vi "Programmer.vi"(0 "Number of Repetitions":i32, 1 "Action":T7=enum."Execute Programmer", 5 "Step Array":T5[](array[typedef])=[{"Airflow (CFM)"={"Setpoint"=0.0, "Stability Range (±)"=0.0}, "Air Temp (°F)"={"Setpoint"=0.0, "Stability Range (±)"=0.0}, "Glycol Flow (lbm/hr)"={"Setpoint"=0.0, "Stability Range (±)"=0.0}, "Glycol Temp (°F)"={"Setpoint"=0.0, "Stability Range (±)"=0.0}, "Hold Time (min)"=0.0, "Stability Test Time (min)"=0.0, "Stability Timeout (min)"=0.0, "Defrost?"=FALSE}], 9 "ANALOG In":T2, 11 "error in (no error)":errorcluster, 12 "Calc Values In":T3) -> (2 "Defrost?":bool, 3 "Setpoints":T4, 4 "Testing is Active?":bool=TRUE, 6 "Current Step":i32, 8 "Time til Step End":dbl format="%<%H:%M:%S>t", 10 "Programmer State":T1, 14 "Components Stable?":bool[](array[boolean]), 15 "error out":errorcluster)   [LabVIEW 2012]
uses:
  Data Types/Programmer Execution States.ctl
  Data Types/Programmer Step.ctl
  Data Types/Programmer Step References.ctl
  Controls/HXG2_Calculated.ctl
  Controls/HXG2_AnalogIn.ctl
  Data Types/Programmer State.ctl
  Support/Time Based Queue/TimeBasedQueue.lvclass
  HXG2programmer.ctl
panel:
  in  "User Input Cluster":T4
  # "Stability (min)"
  # "Running (min)"
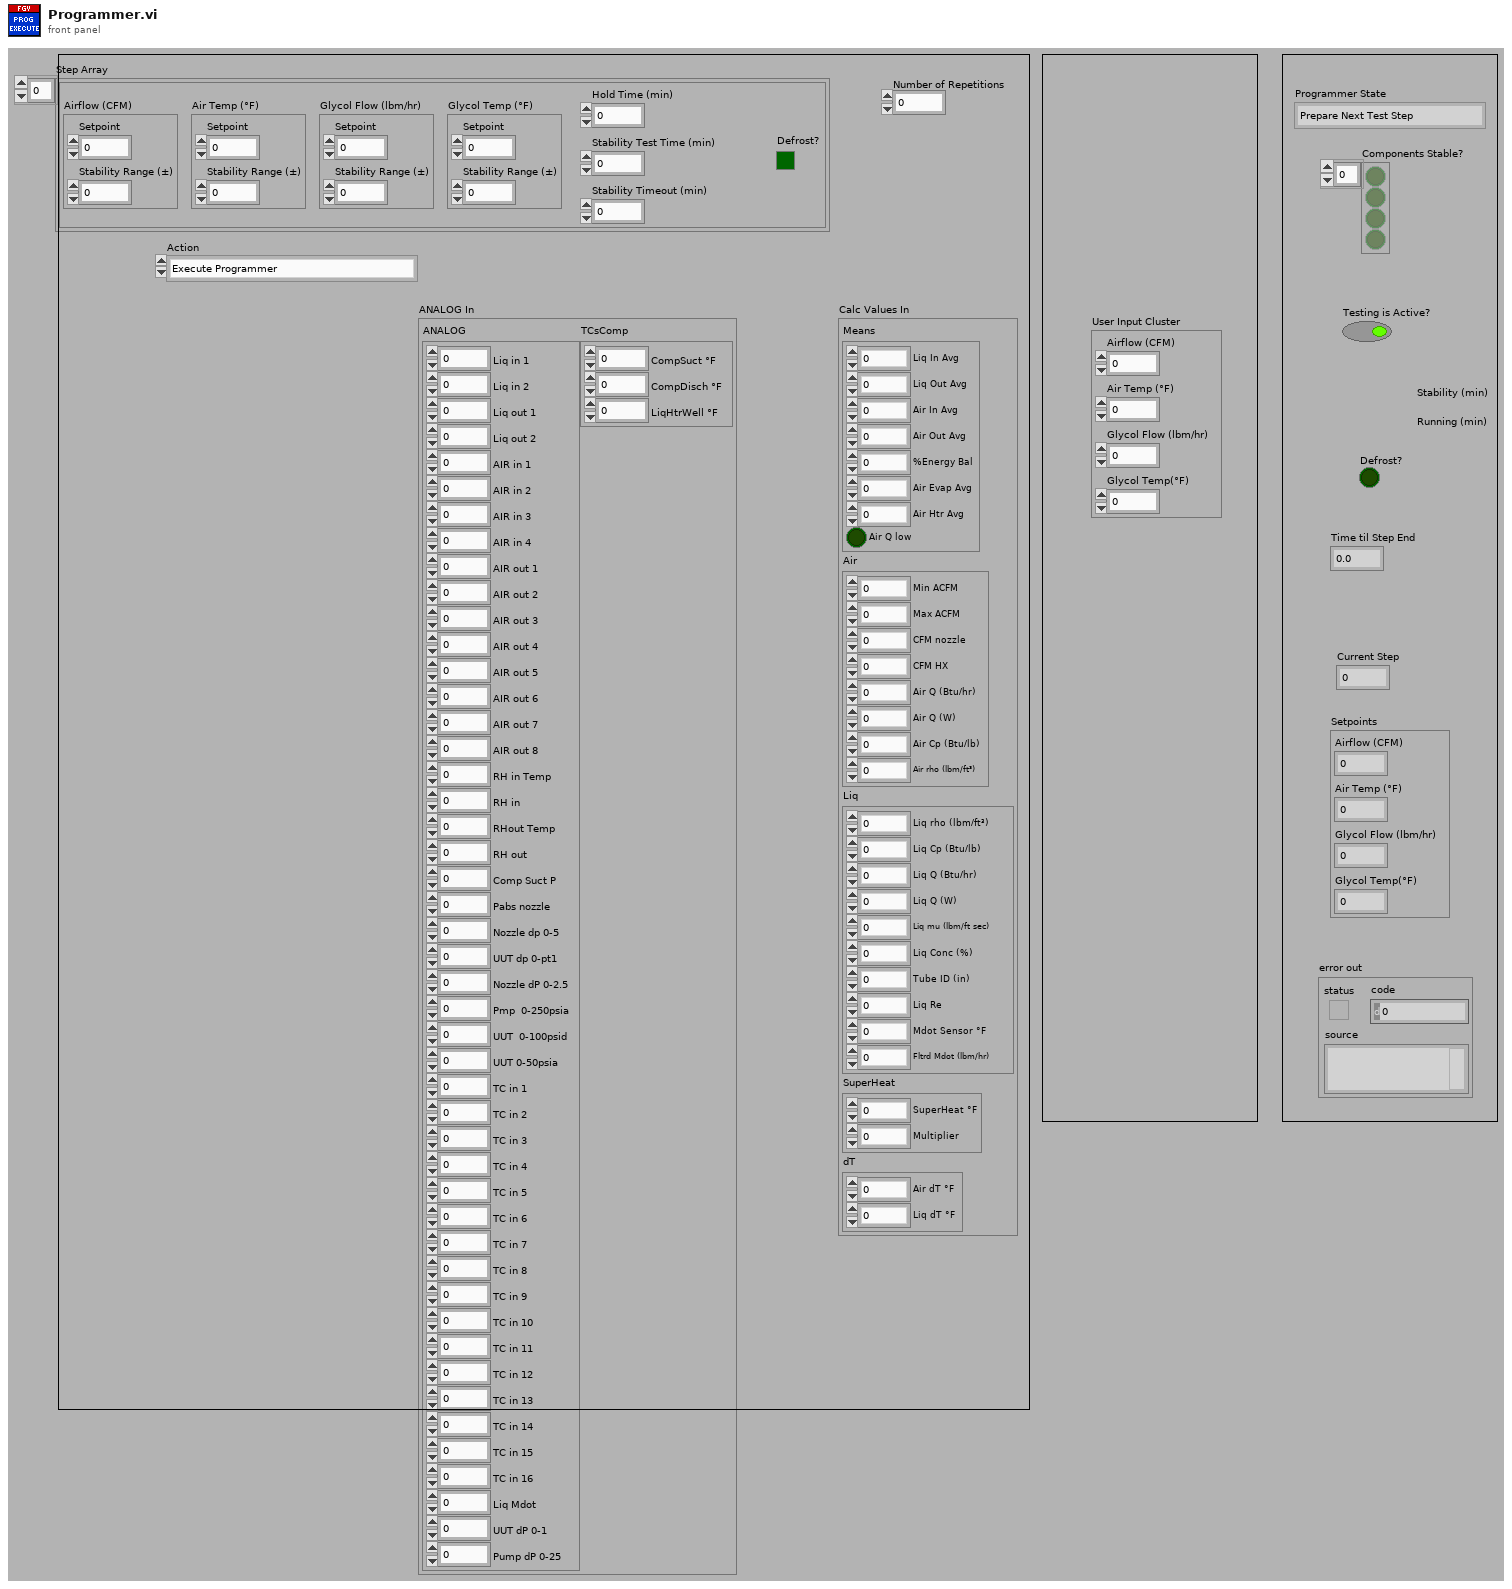
[diagram p1: front panel]
types:
  T1 = typedef "Programmer State.ctl" = enum16{"Prepare Next Test Step", "Stopped", "Running", "Stabilizing"}
  T2 = typedef "HXG2_AnalogIn.ctl" = cluster{"ANALOG":cluster{"Liq in 1":dbl, "Liq in 2":dbl, "Liq out 1":dbl, "Liq out 2":dbl, "AIR in 1":dbl, "AIR in 2":dbl, "AIR in 3":dbl, "AIR in 4":dbl, "AIR out 1":dbl, "AIR out 2":dbl, "AIR out 3":dbl, "AIR out 4":dbl, "AIR out 5":dbl, "AIR out 6":dbl, "AIR out 7":dbl, "AIR out 8":dbl, "RH in Temp":dbl, "RH in":dbl, "RHout Temp":dbl, "RH out":dbl, "Comp Suct P":dbl, "Pabs nozzle":dbl, "Nozzle dp 0-5":dbl, "UUT dp 0-pt1":dbl, "Nozzle dP 0-2.5":dbl, "Pmp  0-250psia":dbl, "UUT  0-100psid":dbl, "UUT 0-50psia":dbl, "TC in 1":dbl, "TC in 2":dbl, "TC in 3":dbl, "TC in 4":dbl, "TC in 5":dbl, "TC in 6":dbl, "TC in 7":dbl, "TC in 8":dbl, "TC in 9":dbl, "TC in 10":dbl, "TC in 11":dbl, "TC in 12":dbl, "TC in 13":dbl, "TC in 14":dbl, "TC in 15":dbl, "TC in 16":dbl, "Liq Mdot":dbl, "UUT dP 0-1":dbl, "Pump dP 0-25":dbl}, "TCsComp":cluster{"CompSuct °F  ":dbl, "CompDisch °F":dbl, "LiqHtrWell °F":dbl}}
  T3 = typedef "HXG2_Calculated.ctl" = cluster{"Means":cluster{"Liq In Avg":dbl, "Liq Out Avg":dbl, "Air In Avg":dbl, "Air Out Avg":dbl, "%Energy Bal":dbl, "Air Evap Avg":dbl, "Air Htr Avg":dbl, "Air Q low":bool}, "Air":cluster{"Min ACFM":dbl, "Max ACFM":dbl, "CFM nozzle":dbl, "CFM HX":dbl, "Air Q (Btu/hr)":dbl, "Air Q (W)":dbl, "Air Cp (Btu/lb)":dbl, "Air rho (lbm/ft³)":dbl}, "Liq":cluster{"Liq rho (lbm/ft³)":dbl, "Liq Cp (Btu/lb)":dbl, "Liq Q (Btu/hr)":dbl, "Liq Q (W)":dbl, "Liq mu (lbm/ft sec)":dbl, "Liq Conc (%)":dbl, "Tube ID (in)":dbl, "Liq Re":dbl, "Mdot Sensor °F":dbl, "Fltrd Mdot (lbm/hr)":dbl}, "SuperHeat":cluster{"SuperHeat °F":dbl, "Multiplier":dbl}, "dT":cluster{"Air dT °F":dbl, "Liq dT °F":dbl}}
  T4 = cluster{"Airflow (CFM)":dbl, "Air Temp (°F)":dbl, "Glycol Flow (lbm/hr)":dbl, "Glycol Temp(°F)":dbl}
  T5 = typedef "Programmer Step.ctl" = cluster{"Airflow (CFM)":T6, "Air Temp (°F)":T6, "Glycol Flow (lbm/hr)":T6, "Glycol Temp (°F)":T6, "Hold Time (min)":dbl, "Stability Test Time (min)":dbl, "Stability Timeout (min)":dbl, "Defrost?":bool}
  T6 = typedef "Programmer Step References.ctl" = cluster{"Setpoint":dbl, "Stability Range (±)":dbl}
  T7 = typedef "Programmer Execution States.ctl" = enum16{"Register Steps", "Initialize", "Start Test Sequence", "Register Data", "Execute Programmer", "Set Number of Repetitions", "Get Current Step Index", "Get Time Until Step Ends"}
  T8 = typedef "HXG2programmer.ctl" = enum16{"Write Refs", "Write Selec", "Write All", "Pass All", "React", "Write Path"}
  T9 = typedef "HXG2_ProgRefs.ctl" = cluster{"Prog. Indicator":refnum<vi>, "Table":refnum<vi>, "Save Button":refnum<vi>, "Duration Ctrl":refnum<vi>, "Run Prog":refnum<vi>}
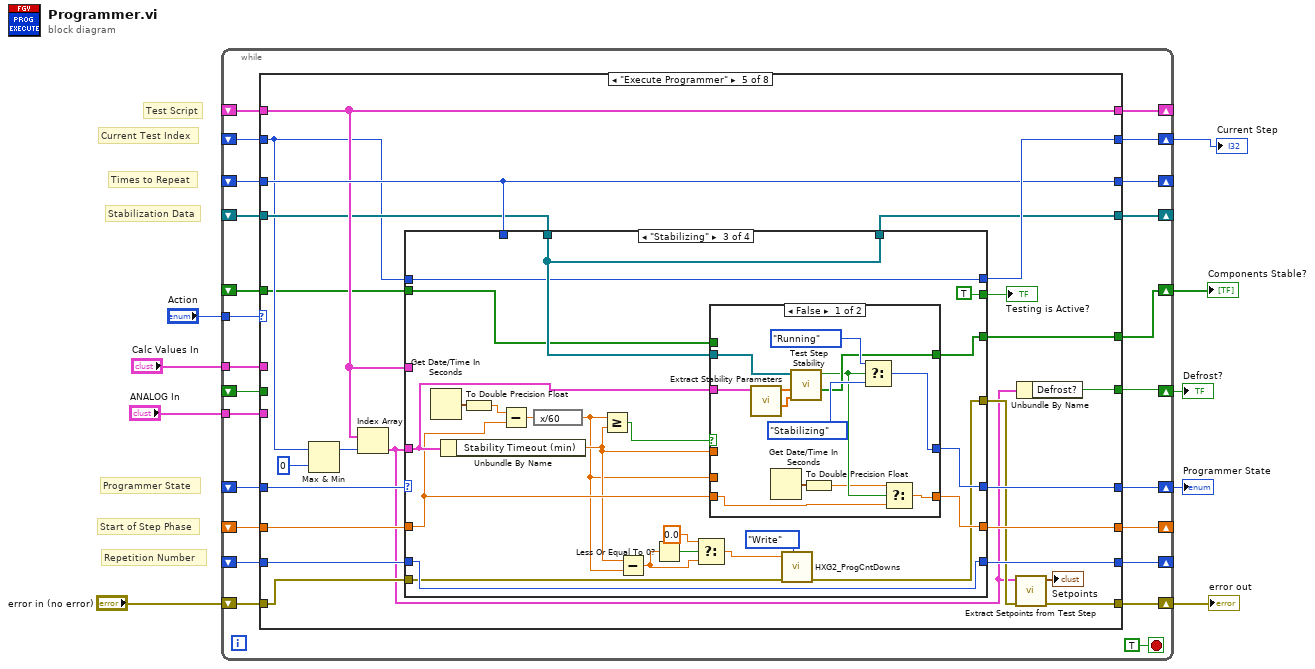
[diagram p0: block diagram]
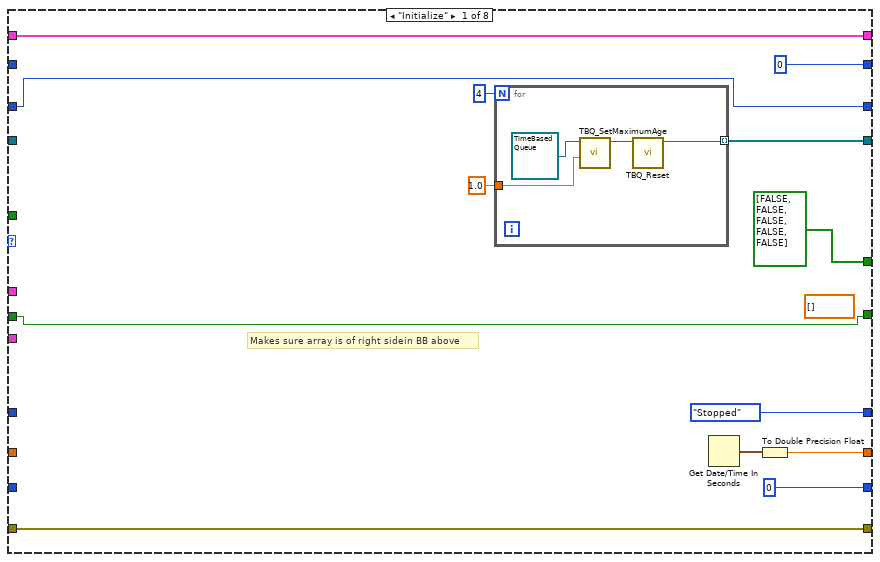
[diagram p2: hidden frame]
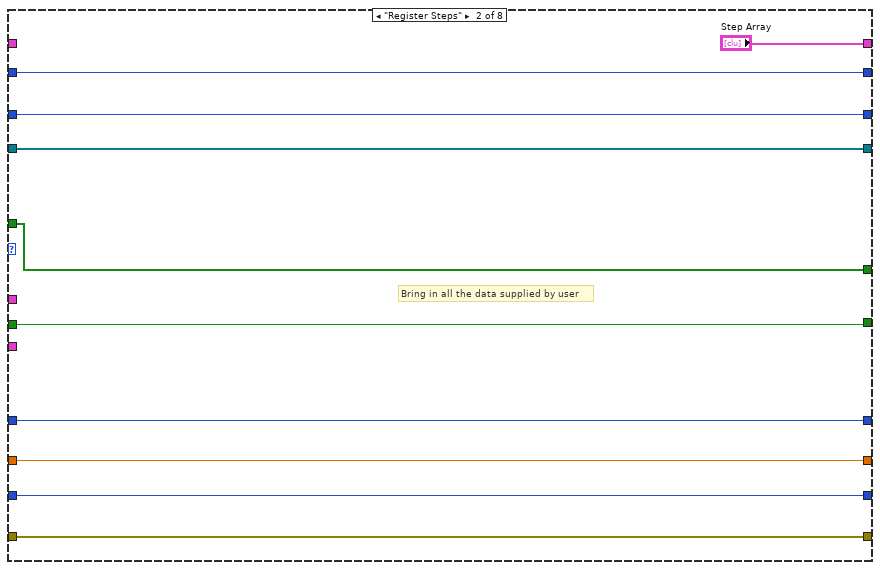
[diagram p3: hidden frame]
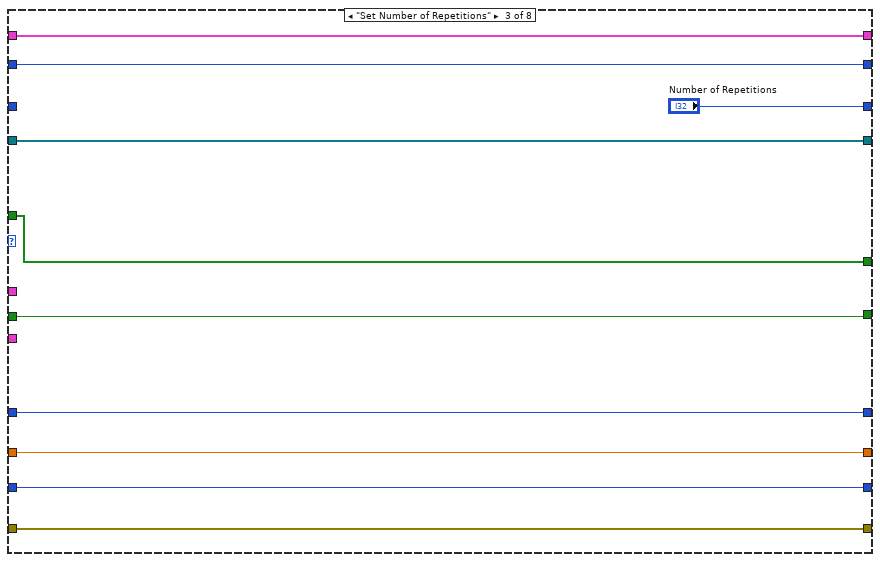
[diagram p4: hidden frame]
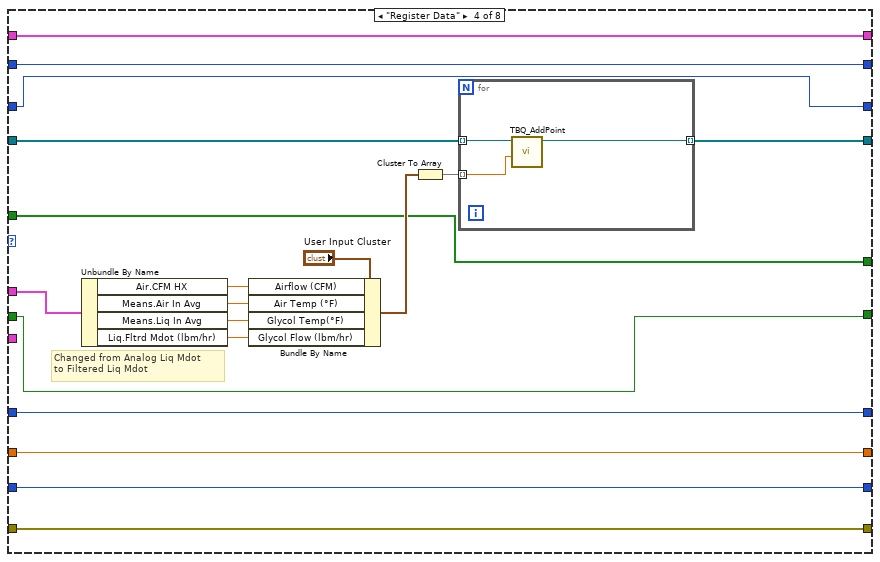
[diagram p5: hidden frame]
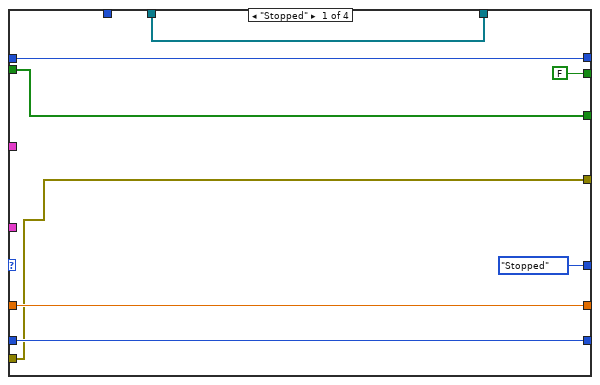
[diagram p6: hidden frame]
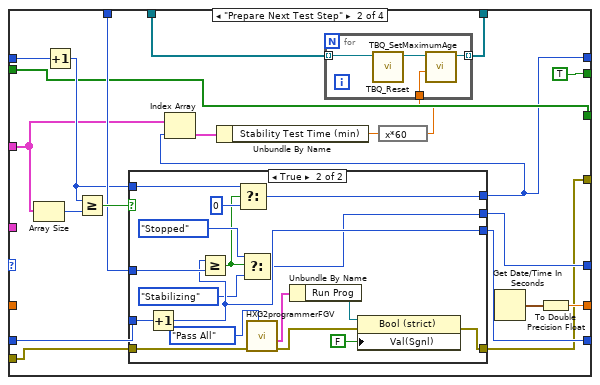
[diagram p7: hidden frame]
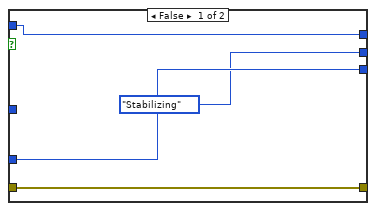
[diagram p8: hidden frame]
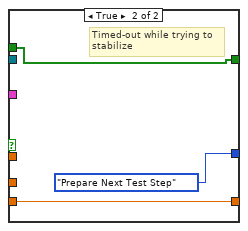
[diagram p9: hidden frame]
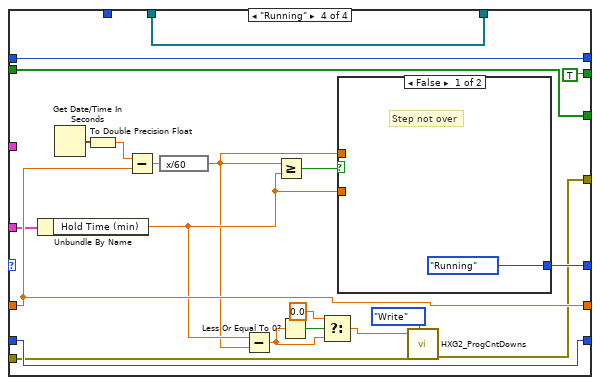
[diagram p10: hidden frame]
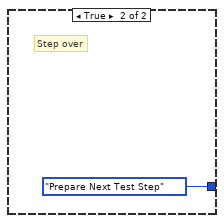
[diagram p11: hidden frame]
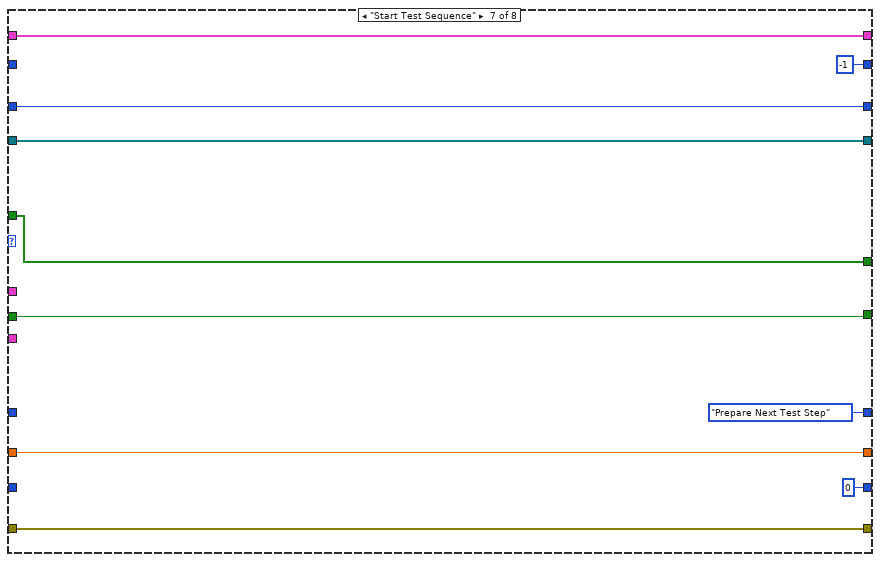
[diagram p13: hidden frame]
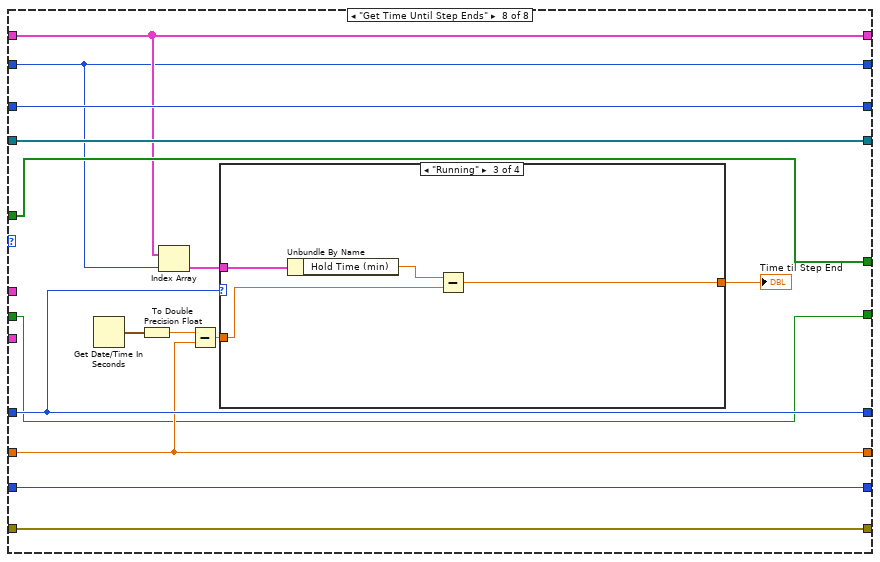
[diagram p14: hidden frame]
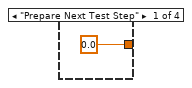
[diagram p15: hidden frame]
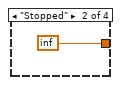
[diagram p16: hidden frame]
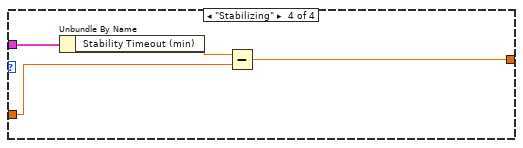
[diagram p17: hidden frame]
diagram:
  # "Repetition Number"
  # "Times to Repeat"
  # "Start of Step Phase"
  # "Programmer State"
  # "Stabilization Data"
  # "Current Test Index"
  # "Test Script"
  n1 = while {
    tunnel: "Action" -> [w33]
    shift-right: [w32] -> _
    shift-left: _ -> [w31]
    shift-right: [w29] -> w2
    shift-left: _ -> [w28]
    shift-right: [w27] -> w8
    shift-left: "error in (no error)" -> [w26]
    shift-right: [w25] -> _
    shift-left: _ -> [w24]
    shift-right: [w23] -> w4
    shift-left: _ -> [w22]
    shift-right: [w21] -> _
    shift-left: _ -> [w20]
    shift-right: [w19] -> _
    shift-left: _ -> [w18]
    shift-right: [w17] -> _
    shift-left: _ -> [w16]
    tunnel: "ANALOG In" -> [w15]
    tunnel: "Calc Values In" -> [w14]
    shift-right: [w13] -> w3
    shift-left: _ -> [w12]
    shift-right: [w11] -> w1
    shift-left: _ -> [w10]
    stop <- TRUE stop-if-true
    n2 = case shown="\"Execute Programmer\"" w33 {
      tunnel: [w42 "Step Array" w70 w89 w106 w241 w251 w256] -> w32
      tunnel: w31 -> [w42 _ w70 w89 w106 w241 w251 w256]
      tunnel: [0 w59 w69 w88 w113 w233 -1 ("f") w255] -> w29
      tunnel: w28 -> [_ w59 w69 w88 w100 w233 _ w255]
      tunnel: [w45 w58 w68 w87 w104 w240 w250 w266] -> w27
      tunnel: w26 -> [w45 w58 w68 w87 w96 w240 w250 w266]
      tunnel: [w44 w57 w67 w84 w102 w239 w249 w265] -> w25
      tunnel: w24 -> [_ w57 w67 w85 w103 w239 w249 w265]
      tunnel: [Programmer_State."Stopped" ("Programmer State") w55 w66 w82 w112 w237 Programmer_State."Prepare Next Test Step" ("Programmer State") w254] -> w23
      tunnel: w22 -> [_ w55 w66 w82 w115 w237 _ w254]
      tunnel: [w40 w56 w65 w83 w111 w238 w248 w253] -> w21
      tunnel: w20 -> [_ w56 w65 w83 w114 w238 w248 w253]
      tunnel: [w38 w54 "Number of Repetitions" w81 w109 w236 w247 w264] -> w19
      tunnel: w18 -> [w38 w54 _ w81 w109 w236 w247 w264]
      tunnel: [0 w53 w63 w80 w108 w235 0 w263] -> w17
      tunnel: w16 -> [_ w53 w63 w80 w110 w235 _ w263]
      tunnel: w15 -> [_ _ _ _ _ _ _ _]
      tunnel: w14 -> [_ _ _ w77 _ _ _ _]
      tunnel: [bool[] [FALSE, FALSE, FALSE, FALSE, FALSE] ("Components Stable?") w52 w62 w73 w98 w234 w243 w262] -> w13
      tunnel: w12 -> [_ w52 w62 w73 w97 w234 w243 w262]
      tunnel: [w34 w51 w61 w71 w93 w232 w242 w252] -> w11
      tunnel: w10 -> [w34 w51 w61 w71 _ w232 w242 w252]
      frame "Initialize" {
        (unwired) dbl[] []
        # "Makes sure array is of right sidein BB above"
        n3 = for {
          N: 4 -> [_]
          tunnel: [w48] -> w44 mode=indexing
          tunnel: 1.0 ("Stability Test Time (min)") -> [w47]
          n4 = call "TBQ_SetMaximumAge.vi"("Maximum Age (s)"=w47, "TimeBasedQueue In"=refnum<class "TimeBasedQueue.lvclass"> refnum ("TimeBasedQueue.lvclass")) -> ("TimeBasedQueue Out"=w49:refnum<class "TimeBasedQueue.lvclass">)  [unwired: 9 in]
          n5 = call "TBQ_Reset.vi"("TimeBasedQueue In"=w49) -> ("TimeBasedQueue Out"=w48:refnum<class "TimeBasedQueue.lvclass">)  [unwired: 10 in]
        }
        n6 = Get Date/Time In Seconds() -> (seconds since 1Jan1904=w41:timestamp)
        n7 = To Double Precision Float(number=w41) -> (double precision float=w40:dbl)
      }
      frame "Register Steps" {
        # "Bring in all the data supplied by user"
      }
      frame "Set Number of Repetitions" {
      }
      frame "Register Data" {
        # "Changed from Analog Liq Mdot\nto Filtered Liq Mdot"
        n8 = Unbundle By Name(w77) -> ("Air.CFM HX"=w76:dbl, "Means.Air In Avg"=w75:dbl, "Means.Liq In Avg"=w74:dbl, "Liq.Fltrd Mdot (lbm/hr)"=w72:dbl)
        n9 = Bundle By Name(cluster="User Input Cluster", "Airflow (CFM)"=w76, "Air Temp (°F)"=w75, "Glycol Temp(°F)"=w74, "Glycol Flow (lbm/hr)"=w72) -> (w79:T4)
        n10 = Cluster To Array(cluster=w79) -> (array=w86:dbl[])
        n11 = for {
          tunnel: w86 -> [w91] mode=indexing
          tunnel: w85 -> [w92] mode=indexing
          tunnel: [w90] -> w84 mode=indexing
          n12 = call "TBQ_AddPoint.vi"("New Data Point"=w91, "TimeBasedQueue In"=w92) -> ("TimeBasedQueue Out"=w90:refnum<class "TimeBasedQueue.lvclass">)  [unwired: 9 in]
        }
      }
      frame "Execute Programmer" {
        n13 = Max & Min(x=w100, y=0) -> (max(x,y)=w99:i32)  [unwired: 1 out]
        n14 = Index Array(array=w106, index=w99) -> (element=w94:T5)
        n15 = case shown="\"Stabilizing\"" w115 {
          tunnel: w103 -> [w118 w130 w192 w219]
          tunnel: [Programmer_State."Stopped" ("Programmer State") w136 w191 w225] -> w112
          tunnel: w114 -> [w120 _ w179 w223]
          tunnel: w94 -> [_ _ w186 w220]
          tunnel: w100 -> [w122 w142 w185 w224]
          tunnel: [w122 w126 w185 w224] -> w113
          tunnel: [w120 w143 w180 w223] -> w111
          tunnel: w110 -> [w123 w139 w184 w222]
          tunnel: w106 -> [_ w133 _ _]
          tunnel: w109 -> [_ w138 _ _]
          tunnel: [w123 w137 w184 w222] -> w108
          tunnel: [FALSE TRUE TRUE TRUE] -> w107
          tunnel: [w118 w129 w192 w219] -> w102
          tunnel: [w117 w128 w182 w218] -> w98
          tunnel: w97 -> [w117 w128 w181 w218]
          tunnel: w96 -> [w116 w125 w175 w212]
          tunnel: [w116 w124 w174 w211] -> w95
          frame "Stopped" {
          }
          frame "Prepare Next Test Step" {
            n16 = Array Size(array=w133) -> (size(s)=w140:i32)
            n17 = Increment(x=w142) -> (x+1=w135:i32)
            n18 = Greater Or Equal?(x=w135, y=w140) -> (x >= y?=w141:bool)
            n19 = case shown="True" w141 {
              tunnel: w139 -> [w152 w169]
              tunnel: w138 -> [_ w168]
              tunnel: [w152 w167] -> w137
              tunnel: [Programmer_State."Stabilizing" ("Programmer State") w166] -> w136
              tunnel: w135 -> [w150 w163]
              tunnel: [w150 w162] -> w126
              tunnel: w125 -> [w149 w154]
              tunnel: [w149 w153] -> w124
              frame False {
              }
              frame True {
                n20 = Increment(x=w169) -> (x+1=w167:i32)
                n21 = Greater Or Equal?(x=w167, y=w168) -> (x >= y?=w160:bool)
                n22 = Select(t=w163, s=w160, f=0) -> (s? t:f=w162:i32)
                n23 = Select(t=Programmer_State."Stopped" ("Programmer State"), s=w160, f=Programmer_State."Stabilizing" ("Programmer State")) -> (s? t:f=w166:T1)
                n24 = call "HXG2programmerFGV.vi"("Programmer Ctrl"=HXG2programmer."Pass All", "error in (no error)"=w154) -> ("error out"=w158:errorcluster, "References Out"=w156:T9)  [unwired: 5 in, 3 out]
                n25 = Unbundle By Name(w156) -> ("Run Prog"=w155:refnum<vi>)
                n26 = property class="Bool (strict)"(reference=w155, error in=w158, "Val(Sgnl)"=FALSE ("Value (Signaling)")) -> (error out=w153:errorcluster)  [unwired: 1 out]
              }
            }
            n27 = Index Array(array=w133, index=w126) -> (element=w132:T5)
            n28 = Unbundle By Name(w132) -> ("Stability Test Time (min)"=w131:dbl)
            n29 = expression code="x*60"(w131) -> (w127:dbl)
            n30 = for {
              tunnel: w127 -> [w147]
              tunnel: w130 -> [w146] mode=indexing
              tunnel: [w145] -> w129 mode=indexing
              n31 = call "TBQ_Reset.vi"("TimeBasedQueue In"=w146) -> ("TimeBasedQueue Out"=w148:refnum<class "TimeBasedQueue.lvclass">)  [unwired: 10 in]
              n32 = call "TBQ_SetMaximumAge.vi"("Maximum Age (s)"=w147, "TimeBasedQueue In"=w148) -> ("TimeBasedQueue Out"=w145:refnum<class "TimeBasedQueue.lvclass">)  [unwired: 9 in]
            }
            n33 = Get Date/Time In Seconds() -> (seconds since 1Jan1904=w144:timestamp)
            n34 = To Double Precision Float(number=w144) -> (double precision float=w143:dbl)
          }
          frame "Stabilizing" {
            n35 = Get Date/Time In Seconds() -> (seconds since 1Jan1904=w190:timestamp)
            n36 = Unbundle By Name(w186) -> ("Stability Timeout (min)"=w172:dbl)
            n37 = To Double Precision Float(number=w190) -> (double precision float=w189:dbl)
            n38 = Subtract(x=w189, y=w179) -> (x-y=w188:dbl)
            n39 = expression code="x/60"(w188) -> (w171:dbl)
            n40 = Greater Or Equal?(x=w171, y=w172) -> (x >= y?=w187:bool)
            n41 = Subtract(x=w172, y=w171) -> (x-y=w177:dbl)
            n42 = Less Or Equal To 0?(x=w177) -> (x <= 0?=w176:bool)
            n43 = Select(t=0.0, s=w176, f=w177) -> (s? t:f=w170:dbl)
            n44 = case shown="False" w187 {
              tunnel: w192 -> [w203 _]
              tunnel: [w202 Programmer_State."Prepare Next Test Step" ("Programmer State")] -> w191
              tunnel: w186 -> [w201 _]
              tunnel: [w198 w207] -> w182
              tunnel: w181 -> [_ w207]
              tunnel: [w196 w206] -> w180
              tunnel: w179 -> [w195 w206]
              tunnel: w171 -> [_ _]
              tunnel: w172 -> [_ _]
              frame False {
                n45 = call "Extract Stability Parameters.vi"("Programmer Step"=w201) -> ("Ranges"=w205:dbl[], "Setpoints"=w204:dbl[])  [unwired: 9 in]
                n46 = Get Date/Time In Seconds() -> (seconds since 1Jan1904=w194:timestamp)
                n47 = call "Test Step Stability.vi"("Ranges"=w205, "Setpoints"=w204, "Array"=w203) -> ("Components Stable?"=w198:bool[], "System Stable?"=w197:bool)  [unwired: 5 in, 2 out]
                n48 = To Double Precision Float(number=w194) -> (double precision float=w193:dbl)
                n49 = Select(t=Programmer_State."Running" ("Programmer State"), s=w197, f=Programmer_State."Stabilizing" ("Programmer State")) -> (s? t:f=w202:T1)
                n50 = Select(t=w193, s=w197, f=w195) -> (s? t:f=w196:dbl)
              }
              frame True {
                # "Timed-out while trying to stabilize"
              }
            }
            n51 = call "HXG2_ProgCntDowns.vi"("FGVctrl"=enum16{"Write", "Pass"}."Write", "error in (no error)"=w175, "Numeric"=w170) -> ("error out"=w174:errorcluster)  [unwired: 7 in, 1 out]
          }
          frame "Running" {
            n52 = Unbundle By Name(w220) -> ("Hold Time (min)"=w210:dbl)
            n53 = Get Date/Time In Seconds() -> (seconds since 1Jan1904=w229:timestamp)
            n54 = To Double Precision Float(number=w229) -> (double precision float=w228:dbl)
            n55 = Subtract(x=w228, y=w223) -> (x-y=w227:dbl)
            n56 = expression code="x/60"(w227) -> (w209:dbl)
            n57 = Subtract(x=w210, y=w209) -> (x-y=w216:dbl)
            n58 = Greater Or Equal?(x=w209, y=w210) -> (x >= y?=w226:bool)
            n59 = Less Or Equal To 0?(x=w216) -> (x <= 0?=w215:bool)
            n60 = Select(t=0.0, s=w215, f=w216) -> (s? t:f=w213:dbl)
            n61 = case shown="False" w226 {
              tunnel: [Programmer_State."Running" ("Programmer State") Programmer_State."Prepare Next Test Step" ("Programmer State")] -> w225
              tunnel: w209 -> [_ _]
              tunnel: w210 -> [_ _]
              frame False {
                # "Step not over"
              }
              frame True {
                # "Step over"
              }
            }
            n62 = call "HXG2_ProgCntDowns.vi"("FGVctrl"=enum16{"Write", "Pass"}."Write", "error in (no error)"=w212, "Numeric"=w213) -> ("error out"=w211:errorcluster)  [unwired: 7 in, 1 out]
          }
        }
        "Testing is Active?" <- w107
        n63 = call "Extract Setpoints from Test Step.vi"("error in (no error)"=w95, "Programmer Step"=w94) -> ("error out"=w104:errorcluster, "Data or Setpoints"=→"Setpoints":T4)  [unwired: 8 in]
        n64 = Unbundle By Name(w94) -> ("Defrost?"=w93:bool)
      }
      frame "Get Current Step Index" {
      }
      frame "Start Test Sequence" {
      }
      frame "Get Time Until Step Ends" {
        n65 = Get Date/Time In Seconds() -> (seconds since 1Jan1904=w260:timestamp)
        n66 = To Double Precision Float(number=w260) -> (double precision float=w261:dbl)
        n67 = Index Array(array=w256, index=w255) -> (element=w258:T5)
        n68 = Subtract(x=w261, y=w253) -> (x-y=w259:dbl)
        n69 = case shown="\"Running\"" w254 {
          tunnel: [0.0 inf w269 w273] -> w257
          tunnel: w258 -> [_ _ w272 w276]
          tunnel: w259 -> [_ _ w270 w274]
          frame "Prepare Next Test Step" {
          }
          frame "Stopped" {
          }
          frame "Running" {
            n70 = Unbundle By Name(w272) -> ("Hold Time (min)"=w271:dbl)
            n71 = Subtract(x=w271, y=w270) -> (x-y=w269:dbl)
          }
          frame "Stabilizing" {
            n72 = Unbundle By Name(w276) -> ("Stability Timeout (min)"=w275:dbl)
            n73 = Subtract(x=w275, y=w274) -> (x-y=w273:dbl)
          }
        }
        "Time til Step End" <- w257
      }
    }
  }
  "error out" <- w8
  "Programmer State" <- w4
  "Components Stable?" <- w3
  "Current Step" <- w2
  "Defrost?" <- w1
